vi "h5_write_attributes.vi"(7 "object name":string, 8 "error in":errorcluster, 10 "attributes":variant, 11 "h5 ref":T1 format="%.0x") -> (0 "error out":errorcluster, 3 "dup h5 ref":T1 format="%.0x")   [LabVIEW 2015]
uses:
  <vilib>/addons/h5labview2/base/hid_t.ctl
  <vilib>/addons/h5labview2/attrib/H5A.lvlib
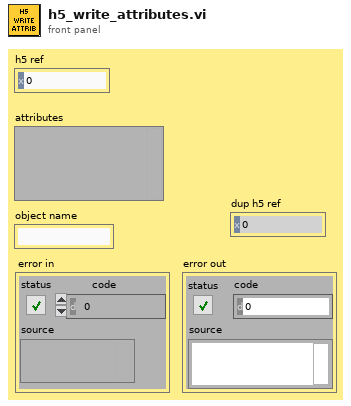
[diagram p1: front panel]
types:
  T1 = typedef "hid_t.ctl" = i32
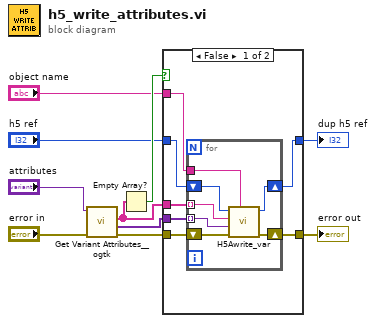
[diagram p0: block diagram]
diagram:
  n1 = call <userlib>:"Get Variant Attributes__ogtk.vi"("error in"="error in", "Variant"="attributes") -> ("error out"=w9:errorcluster, "value(s)"=w10:variant[], "names"=w8:string[])  [unwired: 2 in, 1 out]
  n2 = Empty Array?(array=w8) -> (empty?=w7:bool)
  n3 = case shown="False" w7 {
    tunnel: w8 -> [w17 _]
    tunnel: w10 -> [w16 _]
    tunnel: "h5 ref" -> [w15 w26]
    tunnel: w9 -> [w14 w25]
    tunnel: [w13 w25] -> w1
    tunnel: "object name" -> [w12 _]
    tunnel: [w11 w26] -> w4
    frame False {
      n4 = for {
        tunnel: w17 -> [w24] mode=indexing
        tunnel: w16 -> [w23] mode=indexing
        shift-right: [w20] -> w13
        shift-left: w14 -> [w21]
        shift-right: [w19] -> w11
        shift-left: w15 -> [w22]
        tunnel: w12 -> [w18]
        n5 = call <vilib>:"H5Awrite_var.vi"("object name"=w18, "error in (no error)"=w21, "data"=w23, "attrib name"=w24, "ref in"=w22) -> ("error out"=w20:errorcluster, "ref out"=w19:T1)  [unwired: 4 in, 1 out]
      }
    }
    frame True {
    }
  }
  "dup h5 ref" <- w4
  "error out" <- w1
